vi "Power Consumption.vi"() -> ()   [LabVIEW 2020]
uses:
  <vilib>/regexp/Match Regular Expression.xnode
panel:
  out "Power":u32
  out "Epsilon":u32
  out "Gamma":u32
  in  "Input":string="110011110101\n110011100010\n010100011010\n011001100000\n010011011101\n011110111000\n111111000100\n000100010001\n101101010011\n100101101100\n001111011010\n011111111101\n010111000000\n000011101000\n100101010010\n010011000010\n000011000000\n111100110010\n100100101110\n110000110100\n011110010000\n010101000000\n001000110001\n010111000100\n110111010100\n011001110110\n110001001101\n001101010010\n110111110100\n100111110111\n001001110010\n001100011111\n001111110010\n100111000111\n101111100001\n011100001100\n000000000111\n101111110001\n110111001101\n101111011010\n100101001111\n011101111111\n101101010101\n011011111000\n011100101001\n001101010100\n00..."
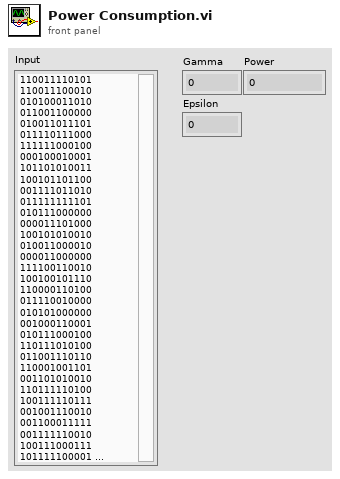
[diagram p1: front panel]
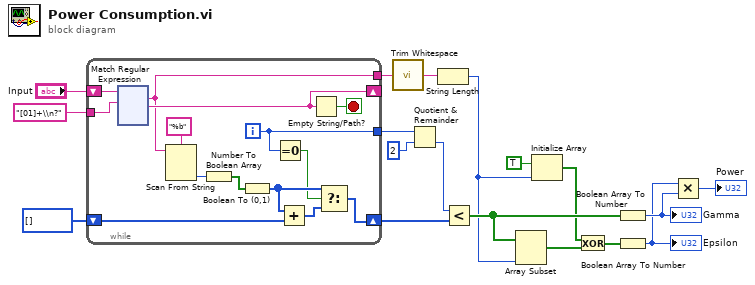
[diagram p0: block diagram]
diagram:
  n1 = while {
    shift-right: [w29] -> _
    shift-left: "Input" -> [w32]
    tunnel: "[01]+\\n?" -> [w31]
    shift-right: [w23] -> w12
    shift-left: i32[] [] -> [w25]
    tunnel: [w21] -> w15
    tunnel: [w19] -> w6
    i -> [w21]
    stop <- w30 stop-if-true
    n2 = xnode "Match Regular Expression"("input string"=w32, "regular expression"=w31) -> ("whole match"=w19:string, "after match"=w29:string)  [unwired: 4 in, 3 out]
    n3 = Scan From String(format string="%b", input string=w19) -> (output 1=w27:i32)  [unwired: 3 in, 3 out]
    n4 = Number To Boolean Array(number=w27) -> (Boolean array=w20:bool[])
    n5 = Boolean To (0,1)(Boolean=w20) -> (0, 1=w26:i16[])
    n6 = Equal To 0?(x=w21) -> (x = 0?=w22:bool)
    n7 = Add(x=w26, y=w25) -> (x+y=w24:i32[])
    n8 = Empty String/Path?(string/path=w29) -> (empty?=w30:bool)
    n9 = Select(t=w26, s=w22, f=w24) -> (s? t:f=w23:i32[])
  }
  n10 = call <vilib>:"Trim Whitespace.vi"("string"=w6) -> ("trimmed string"=w5:string)  [unwired: 1 in]
  n11 = Quotient & Remainder(x=w15, y=2) -> (floor(x/y)=w11:i32)  [unwired: 1 out]
  n12 = String Length(string=w5) -> (length=w4:i32)
  n13 = Less?(x=w11, y=w12) -> (x < y?=w10:bool[])
  n14 = Array Subset(array=w10, length=w4) -> (w9:bool[])  [unwired: 1 in]
  n15 = Initialize Array(TRUE, w4) -> (w8:bool[])
  n16 = Exclusive Or(1:w9, 2:w8) -> (0:w7:bool[])
  n17 = Boolean Array To Number(Boolean array=w10) -> (number=w3:u32)
  "Gamma" <- w3
  n18 = Boolean Array To Number(Boolean array=w7) -> (number=w2:u32)
  "Epsilon" <- w2
  n19 = Multiply(x=w2, y=w3) -> (x*y=→"Power":u32)
